vi "NR_RateMatch.vi"(0 "PA":path, 1 "coded_data":dbl[][](array[numeric]), 2 "C":dbl, 3 "I_LBRM":dbl, 4 "error in (no error)":errorcluster caption="错误输入（无错误）", 5 "Qm":dbl, 6 "LDPC_base_graph":dbl, 7 "DMRS_symbol":dbl, 9 "Nsym_slot":dbl, 10 "Zc":dbl, 11 "prb_num":dbl, 12 "vnum":dbl, 13 "rvid":dbl) -> (14 "rm_data":dbl[][](array[numeric]), 15 "rm_len":dbl[](array[numeric]), 18 "error out":errorcluster caption="错误输出")   [LabVIEW 2015]
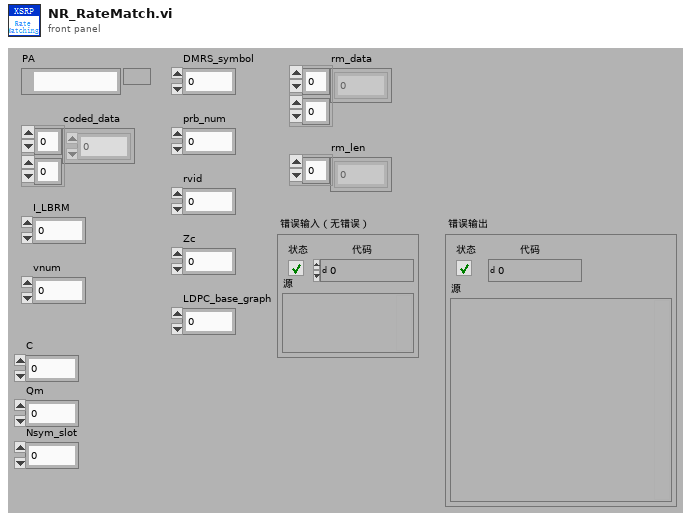
[diagram p1: front panel]
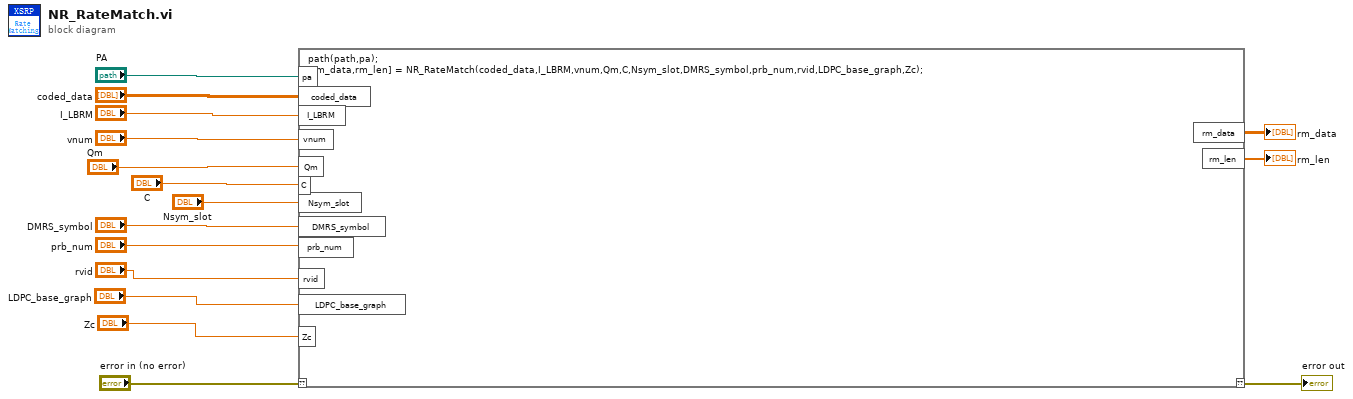
[diagram p0: block diagram]
diagram:
  n1 = script code="path(path,pa);\n[rm_data,rm_len] = NR_RateMatch(coded_data,I_LBRM,vnum,Qm,C,Nsym_slot,DMRS_symbol,prb_num,rvid,LDPC_base_graph,Zc);"("??"="error in (no error)", "pa"="PA", "coded_data"="coded_data", "I_LBRM"="I_LBRM", "vnum"="vnum", "Nsym_slot"="Nsym_slot", "DMRS_symbol"="DMRS_symbol", "prb_num"="prb_num", "rvid"="rvid", "LDPC_base_graph"="LDPC_base_graph", "Zc"="Zc", "C"="C", "Qm"="Qm") -> ("??"=→"error out":errorcluster, "rm_data"=→"rm_data":dbl[][], "rm_len"=→"rm_len":dbl[])
